vi "Send and Forget Data Response.vi"(8 "error in (no error)":errorcluster, 11 "Request Reply Core in":refnum<class "Request Reply Core.lvclass">) -> (0 "error out":errorcluster, 3 "Data":refnum<class "Data.lvclass">)   [LabVIEW 2020, in "Publisher.lvlib" / "Request Reply Core.lvclass"]
doc: "Data generated from the response core when a message is sent as 'Send and Forget'.\n\nThis implementation returns a U32 class with the Request ID."
uses:
  Request Reply Core.lvclass
  PPL/HDH.Data.Generic.lvlibp/Data.lvclass
  Request Reply Core.lvclass/Request Reply Core.ctl
  PPL/HDH.Data.Generic.lvlibp/Generic Data/U32/U32.lvclass
  C:/Current projects/WS/PPL/HDH.Data.Generic.lvlibp/Data.lvclass
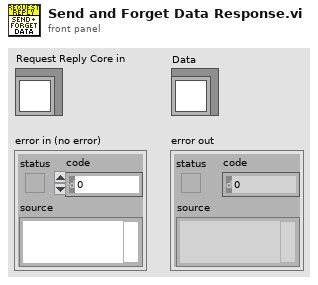
[diagram p1: front panel]
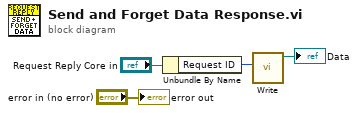
[diagram p0: block diagram]
diagram:
  n1 = Unbundle By Name("Request Reply Core in") -> ("Request ID"=w3:u32)
  n2 = call "Write.vi"("U32"=w3) -> ("U32 out"=→"Data":refnum<class "U32.lvclass">)  [unwired: 10 in]
  "error out" <- "error in (no error)"
